vi "Climb_Solenoid.vi"(8 "Left Bottom Right":bool, 9 "Left Bottom Left":bool, 10 "Left Top Left":bool, 11 "Left Top Right":bool) -> ()   [LabVIEW 2020]
uses:
  <vilib>/Rock Robotics/WPI/Solenoid/WPI_SolenoidValue.ctl
  <vilib>/Rock Robotics/WPI/Solenoid/WPI_SolenoidSetEnum.vi
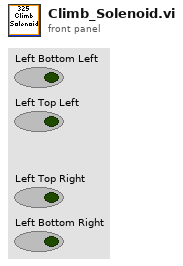
[diagram p1: front panel]
types:
  T1 = typedef "WPI_SolenoidValue.ctl" = enum16{"Off", "On", "Forward", "Reverse"}
  T2 = typedef "WPI_SolenoidDevRef.ctl" = cluster{"DevStatus":errorcluster, "Pneumatics Control Module":u8, "Forward Solenoid Channel":T3, "Reverse Solenoid Channel":T3}
  T3 = typedef "WPI_SolenoidChannel.ctl" = enum8{"Solenoid 0", "Solenoid 1", "Solenoid 2", "Solenoid 3", "Solenoid 4", "Solenoid 5", "Solenoid 6", "Solenoid 7", "Solenoid 8", "Solenoid 9", "Solenoid 10", "Solenoid 11", "Solenoid 12", "Solenoid 13", "Solenoid 14", "Solenoid 15", "Invalid"}
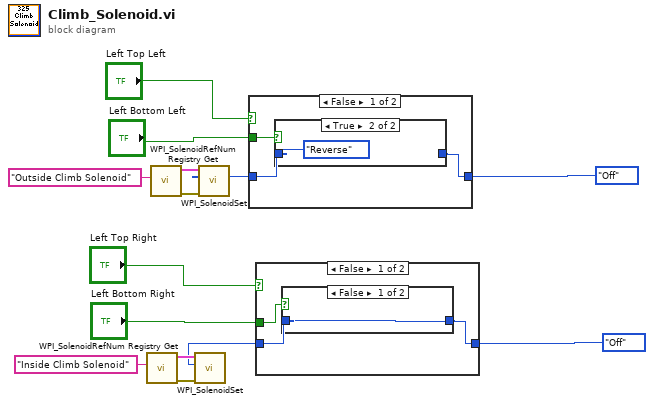
[diagram p0: block diagram]
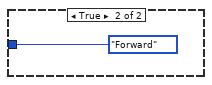
[diagram p3: hidden frame]
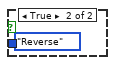
[diagram p4: hidden frame]
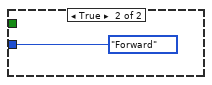
[diagram p5: hidden frame]
diagram:
  n1 = call <vilib>:"WPI_SolenoidRefNum Registry Get.vi"("refnum name"="Inside Climb Solenoid") -> ("error out"=w11:errorcluster, "SolenoidDevRef"=w10:T2)  [unwired: 9 in]
  n2 = call <vilib>:"WPI_SolenoidRefNum Registry Get.vi"("refnum name"="Outside Climb Solenoid") -> ("error out"=w14:errorcluster, "SolenoidDevRef"=w13:T2)  [unwired: 9 in]
  n3 = case shown="False" "Left Top Left" {
    tunnel: [w16 WPI_SolenoidValue."Forward" ("inside climb start")] -> w5
    tunnel: WPI_SolenoidValue."Off" ("inside climb start") -> [w17 _]
    tunnel: "Left Bottom Left" -> [w15 _]
    frame False {
      n4 = case shown="True" w15 {
        tunnel: w17 -> [w18 _]
        tunnel: [w18 WPI_SolenoidValue."Reverse" ("inside climb start")] -> w16
        frame False {
        }
        frame True {
        }
      }
    }
    frame True {
    }
  }
  n5 = call-poly <vilib>:"WPI_SolenoidSet.vi"("error in (no error)"=w14, "Value"=w5, "SolenoidDevRef"=w13) -> ()  [unwired: 7 in, 2 out]
  n6 = case shown="False" "Left Top Right" {
    tunnel: [w22 WPI_SolenoidValue."Forward" ("inside climb start")] -> w8
    tunnel: WPI_SolenoidValue."Off" ("inside climb start") -> [w23 _]
    tunnel: "Left Bottom Right" -> [w21 _]
    frame False {
      n7 = case shown="False" w21 {
        tunnel: w23 -> [w24 _]
        tunnel: [w24 WPI_SolenoidValue."Reverse" ("inside climb start")] -> w22
        frame False {
        }
        frame True {
        }
      }
    }
    frame True {
    }
  }
  n8 = call-poly <vilib>:"WPI_SolenoidSet.vi"("error in (no error)"=w11, "Value"=w8, "SolenoidDevRef"=w10) -> ()  [unwired: 7 in, 2 out]
